vi "filter_test1.vi"() -> ()   [LabVIEW 2021]
panel:
  in  "Numeric":i32
  in  "reset":bool
  out "Waveform Chart":dbl(graph)
  in  "stop":bool
  in  "s":bool
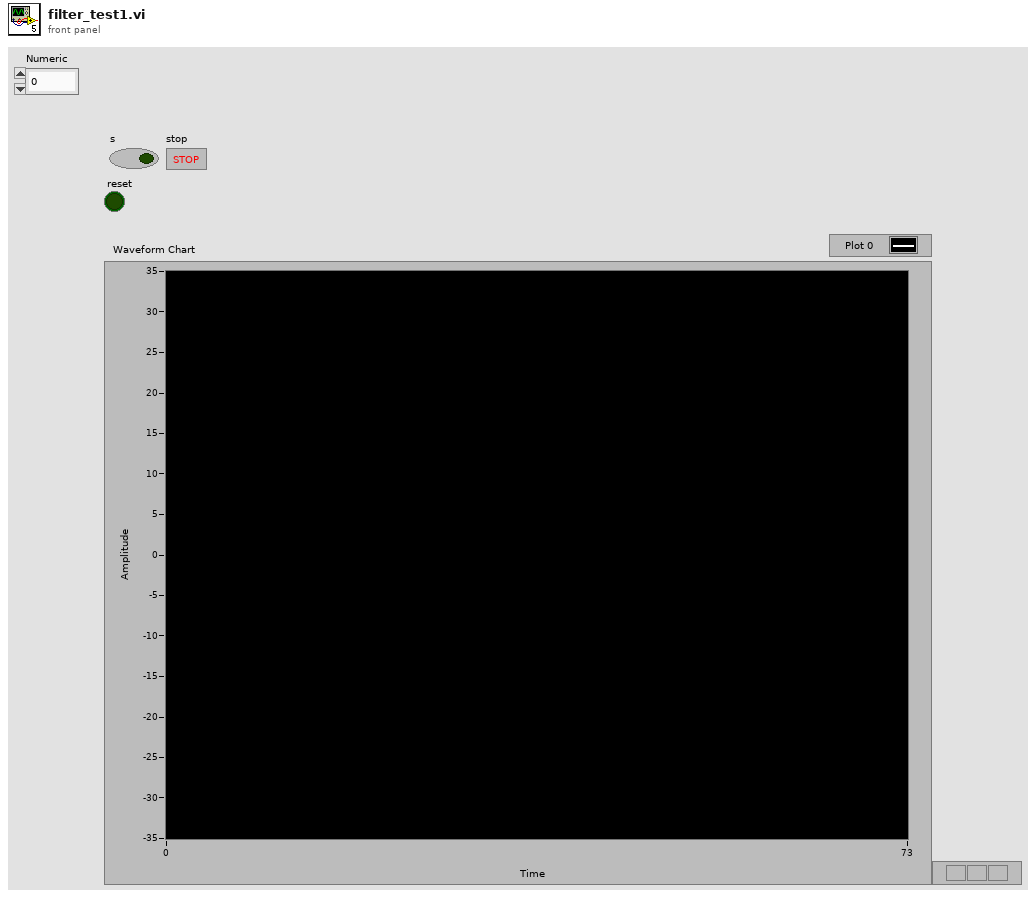
[diagram p1: front panel]
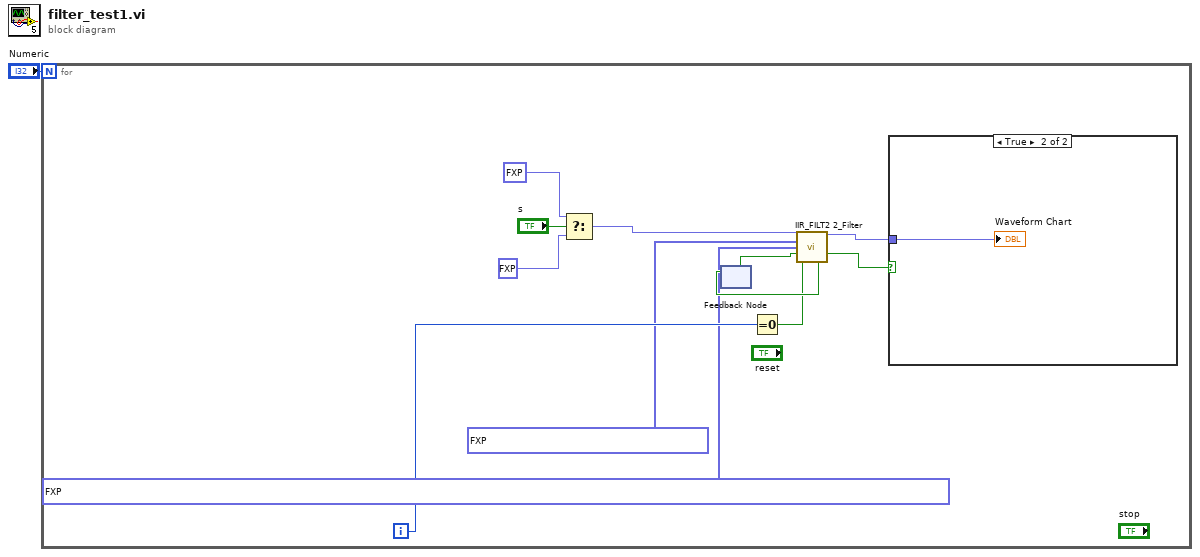
[diagram p0: block diagram]
diagram:
  n1 = for {
    N: "Numeric" -> [_]
    i -> [w4]
    n2 = Select(t=fxp<+/-,16,1> 0.5 ("input data"), s="s", f=fxp<+/-,16,1> 0.0 ("input data")) -> (s? t:f=w9:fxp<+/-,16,1>)
    n3 = feedback #1() -> (w12:bool)  [unwired: 1 in]
    n4 = Equal To 0?(x=w4) -> (x = 0?=w5:bool)
    n5 = call "IIR_FILT2 2_Filter.vi"("input data"=w9, "A"=fxp<+/-,24,2>[] [-1.9955599308013916, 0.9955670833587646], "B"=fxp<+/-,24,-16>[] [2.4619303076178767e-06, 4.923859705741052e-06, 2.4619303076178767e-06], "input valid"=w12, "reset"=w5) -> ("output data"=w7:fxp<+/-,16,6>, "output valid"=w6:bool, "ready for input"=w13:bool)  [unwired: 8 in]
    n6 = feedback-in #1(w13) -> ()
    n7 = case shown="True" w6 {
      tunnel: w7 -> [_ w14]
      frame False {
      }
      frame True {
        "Waveform Chart" <- w14
      }
    }
  }
